vi "ManagerOpen.vi"(8 "error in":errorcluster) -> (0 "error out":errorcluster, 3 "Manager ID":u64 caption="Phidget ID")   [LabVIEW 2012, in "Phidget Manager.lvlib"]
doc: "${Accelerometer:OpenHeader}"
uses:
  <instrlib>/Phidgets/Phidget Manager/Phidget Manager.lvlib
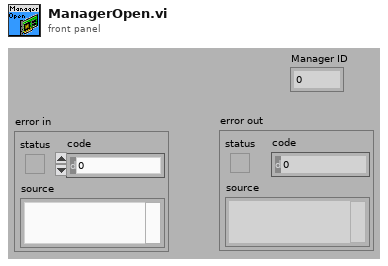
[diagram p1: front panel]
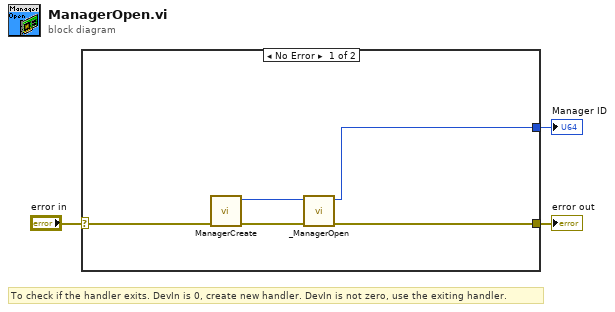
[diagram p0: block diagram]
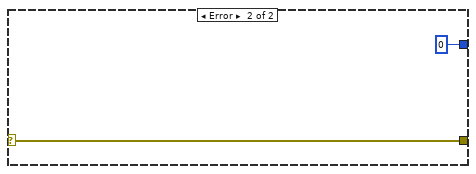
[diagram p2: hidden frame]
diagram:
  # "To check if the handler exits. DevIn is 0, create new handler. DevIn is not zero, use the exiting handler."
  n1 = case shown="No Error" "error in" {
    selector: "error in" -> [w8 w10]
    tunnel: [w6 w10] -> w2
    tunnel: [w5 0 ("Device Out")] -> w1
    frame No Error {
      n2 = call <instrlib>:"ManagerCreate.vi"("error in"=w8) -> ("error out"=w7:errorcluster, "Device Out"=w4:u64)  [unwired: 9 in]
      n3 = call <instrlib>:"_ManagerOpen.vi"("error in"=w7, "Device In"=w4) -> ("error out"=w6:errorcluster, "Device Out"=w5:u64)  [unwired: 8 in]
    }
    frame Error {
    }
  }
  "error out" <- w2
  "Manager ID" <- w1
